vi "CreateArgumentParser.vi"(6 "outputs":T1[](array[typedef]), 7 "parser name":string="parser", 8 "error in":errorcluster, 11 "VI Interpreter in":refnum<class "VI Interpreter.lvclass">) -> (0 "error out":errorcluster, 3 "VI Interpreter out":refnum<class "VI Interpreter.lvclass">, 5 "python assignment":string)   [LabVIEW 2014, in "PyConvBD.lvclass"]
uses:
  PyConvBD.lvclass
  VI Interpreter/Classes/VI Interpreter/VI Interpreter.lvclass
  TypeDefs/ConsoleArg_TD.ctl
  VI Interpreter/Classes/VI Interpreter/VI Interpreter.lvclass/VI Interpreter.ctl
  Parsing/ListTypesTD.ctl
  Parsing/Python Functions.lvlib
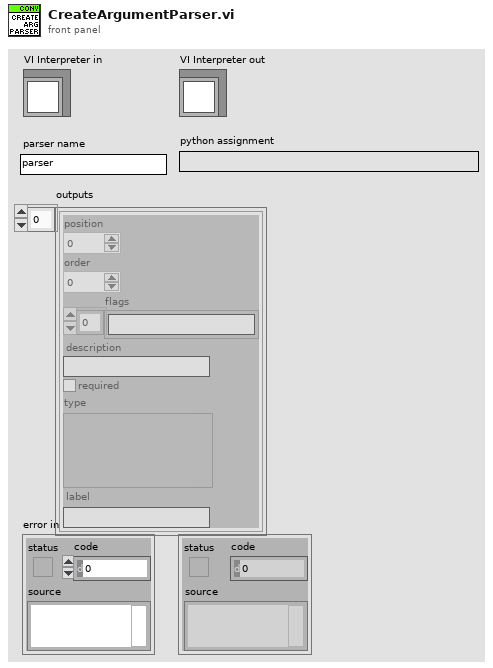
[diagram p1: front panel]
types:
  T1 = typedef "PyConvBD.lvclass/ConsoleArg_TD.ctl" = cluster{"position":i32, "order":i32, "flags":string[], "description":string, "required":bool, "type":variant, "label":string}
  T2 = typedef "Python Functions.lvlib/ListTypesTD.ctl" = enum16{"list", "tuple", "parameter list", "output list", "return values"}
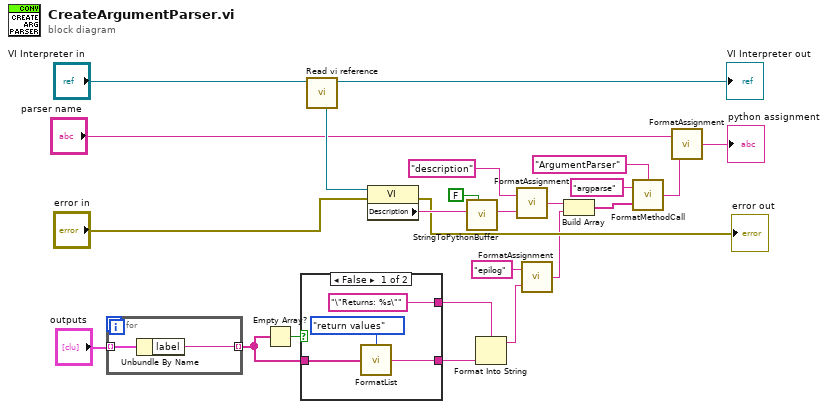
[diagram p0: block diagram]
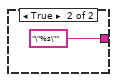
[diagram p2: hidden frame]
diagram:
  n1 = for {
    tunnel: "outputs" -> [w26] mode=indexing
    tunnel: [w25] -> w1 mode=indexing
    n2 = Unbundle By Name(w26) -> ("label"=w25:string)
  }
  n3 = Empty Array?(array=w1) -> (empty?=w7:bool)
  n4 = case shown="False" w7 {
    tunnel: w1 -> [w27 _]
    tunnel: [w29 _] -> w5
    tunnel: ["\"Returns: %s\"" ("format string") "\"%s\"" ("format string")] -> w3
    frame False {
      n5 = call "FormatList.vi"("values"=w27, "type"=ListTypesTD."return values") -> ("python object"=w29:string)
    }
    frame True {
    }
  }
  n6 = call "Read vi reference.vi"("VI Interpreter in"="VI Interpreter in") -> ("VI Interpreter out"=→"VI Interpreter out":refnum<class "VI Interpreter.lvclass">, "vi reference"=w23:refnum<vi>)  [unwired: 7 in]
  n7 = property class="VI"(reference=w23, error in="error in") -> (error out=→"error out":errorcluster, "Description"=w21:string)  [unwired: 1 out]
  n8 = call "StringToPythonBuffer.vi"("Buffer"=FALSE, "string"=w21) -> ("python string"=w19:string)  [unwired: 7 in]
  n9 = Format Into String(format string=w3, w5) -> (resulting string=w4:string)  [unwired: 2 in, 1 out]
  n10 = call "FormatAssignment.vi"("value"=w19, "name"="description") -> ("python assignment"=w17:string)
  n11 = call "FormatAssignment.vi"("value"=w4, "name"="epilog") -> ("python assignment"=w6:string)
  n12 = Build Array(w17, w6) -> (w16:string[])
  n13 = call "FormatMethodCall.vi"("method"="ArgumentParser", "parameters"=w16, "object"="argparse") -> ("python object"=w15:string)
  n14 = call "FormatAssignment.vi"("value"=w15, "name"="parser name") -> ("python assignment"=→"python assignment":string)
